vi "detector_acquire_generic_data.vi"(8 "error in (no error)":errorcluster, 11 "picoharp in":refnum<class "picoharp.lvclass">) -> (0 "error out":errorcluster, 2 "image_data":T1, 3 "picoharp out":refnum<class "picoharp.lvclass">)   [LabVIEW 2015, in "picoharp.lvclass"]
uses:
  picoharp.lvclass
  Experiment/experiment_panel/2d_scan/detector_data_tdef.ctl
  picoharp.lvclass/picoharp.ctl
  <vilib>/Analysis/baseanly.llb/Mean (DBL).vi
  <vilib>/Analysis/NI_AALBase.lvlib
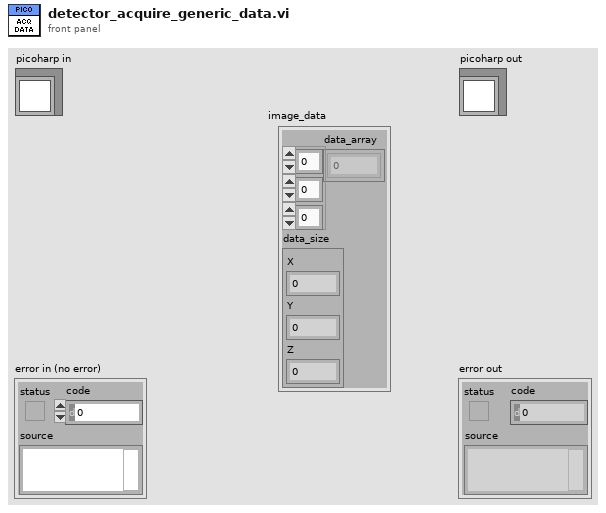
[diagram p1: front panel]
types:
  T1 = typedef "detector_data_tdef.ctl" = cluster{"data_array":dbl[][][], "data_size":cluster{"X":i32, "Y":i32, "Z":i32}}
  T2 = typedef "hydraharp_count_rates.ctl" = cluster{"channel_rates":i32[], "sync_rate":i32}
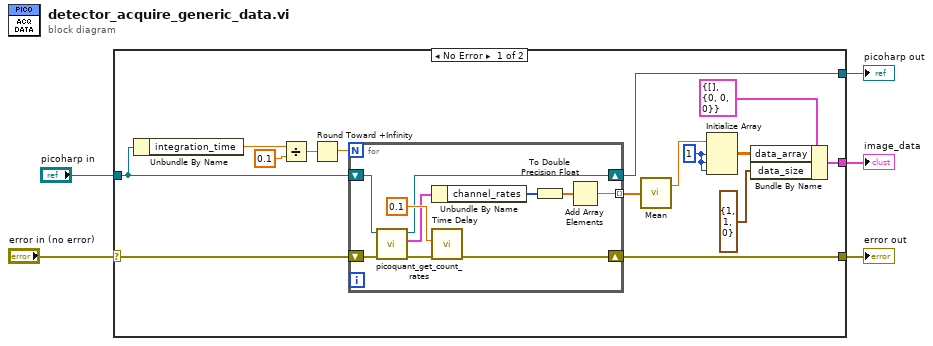
[diagram p0: block diagram]
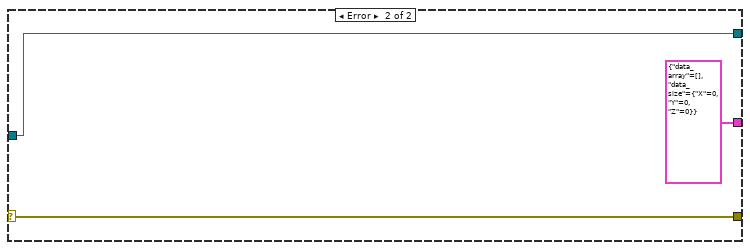
[diagram p2: hidden frame]
diagram:
  n1 = case shown="No Error" "error in (no error)" {
    selector: "error in (no error)" -> [w16 w33]
    tunnel: "picoharp in" -> [w15 w32]
    tunnel: [w14 w33] -> w3
    tunnel: [w7 T1 {"data_array"=[], "data_size"={"X"=0, "Y"=0, "Z"=0}} ("image_data")] -> w2
    tunnel: [w6 w32] -> w1
    frame No Error {
      w13 = 1 ("dimension size")
      n2 = Unbundle By Name(w15) -> ("integration_time"=w18:dbl)
      n3 = Divide(x=w18, y=0.1) -> (x/y=w19:dbl)
      n4 = Round Toward +Infinity(x=w19) -> (ceil(x): smallest int >= x=w17:dbl)
      n5 = for {
        N: w17 -> [_]
        shift-right: [w27] -> w14
        shift-left: w16 -> [w29]
        shift-right: [w25] -> w6
        shift-left: w15 -> [w26]
        tunnel: [w21] -> w11 mode=indexing
        n6 = call-dynamic "picoquant_get_count_rates.vi"("error in (no error)"=w29, "picoharp in"=w26) -> ("error out"=w28:errorcluster, "count_rates"=w22:T2, "picoharp out"=w25:refnum<class "picoharp.lvclass">)  [unwired: 7 in]
        n7 = Unbundle By Name(w22) -> ("channel_rates"=w24:i32[])
        n8 = call "Time Delay"("error in (no error)"=w28, "Delay Time (s)"=0.1) -> ("error out"=w27:errorcluster)  [unwired: 9 in]
        n9 = To Double Precision Float(number=w24) -> (double precision float=w23:dbl[])
        n10 = Add Array Elements(numeric array=w23) -> (sum=w21:dbl)
      }
      n11 = call-poly <vilib>:"Mean.vi"("X"=w11) -> ("mean"=w12:dbl)  [unwired: 1 out]
      n12 = Initialize Array(w12, w13, w13, w13) -> (w9:dbl[][][])
      n13 = Bundle By Name(cluster=T1 {"data_array"=[], "data_size"={"X"=0, "Y"=0, "Z"=0}} ("image_data"), "data_array"=w9, "data_size"=cluster{"X":i32, "Y":i32, "Z":i32} {"X"=1, "Y"=1, "Z"=0}) -> (w7:T1)
    }
    frame Error {
    }
  }
  "error out" <- w3
  "picoharp out" <- w1
  "image_data" <- w2
